vi "Generation Message Loop.vi"(8 "error in (no error)":errorcluster, 10 "Data Notifier":refnum<notifier>, 11 "Message Queues":T1) -> (0 "error out":errorcluster)   [LabVIEW 2014, in "PLS Generation.lvlib"]
doc: "Message loop for handling messages pertaining to the acquisition of data from the hardware."
uses:
  PLS Generation.lvlib
  support/Message Queue/All Message Queues.ctl
  support/Message Queue/Message Cluster.ctl
  Hardware Configuration.ctl
  Settings/conversion.ctl
  Generation State.ctl
  support/Message Queue/Enqueue Message (Single).vi
  <vilib>/Utility/error.llb/Error Cluster From Error Code.vi
  <vilib>/ErrorRing/Error Ring.xnode
  support/Message Queue/PLS Message Queue.lvlib
  Settings/PLS Settings.lvlib
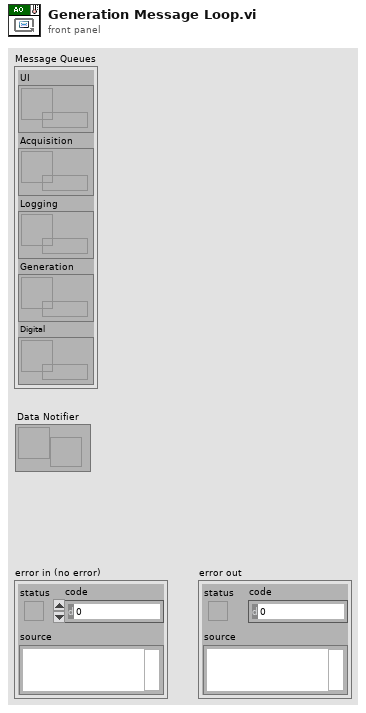
[diagram p1: front panel]
types:
  T1 = typedef "PLS Message Queue.lvlib/All Message Queues.ctl" = cluster{"UI":refnum<queue>, "Acquisition":refnum<queue>, "Logging":refnum<queue>, "Generation":refnum<queue>, "Digital":refnum<queue>}
  T2 = typedef "PLS Generation.lvlib/Hardware Configuration.ctl" = cluster{"AO":cluster{"task name":string, "task_ref":refnum<k21>, "physical channels":tag}, "PID":cluster{"P":dbl, "I":dbl, "D":dbl}, "conversions":cluster{"ao0":T3}, "setpoint":dbl}
  T3 = typedef "PLS Settings.lvlib/conversion.ctl" = cluster{"a":dbl, "b":dbl}
  T4 = typedef "PLS Generation.lvlib/Generation State.ctl" = enum16{"Idle", "Generate"}
  T5 = cluster{"task name":string, "task_ref":refnum<k21>, "physical channels":tag}
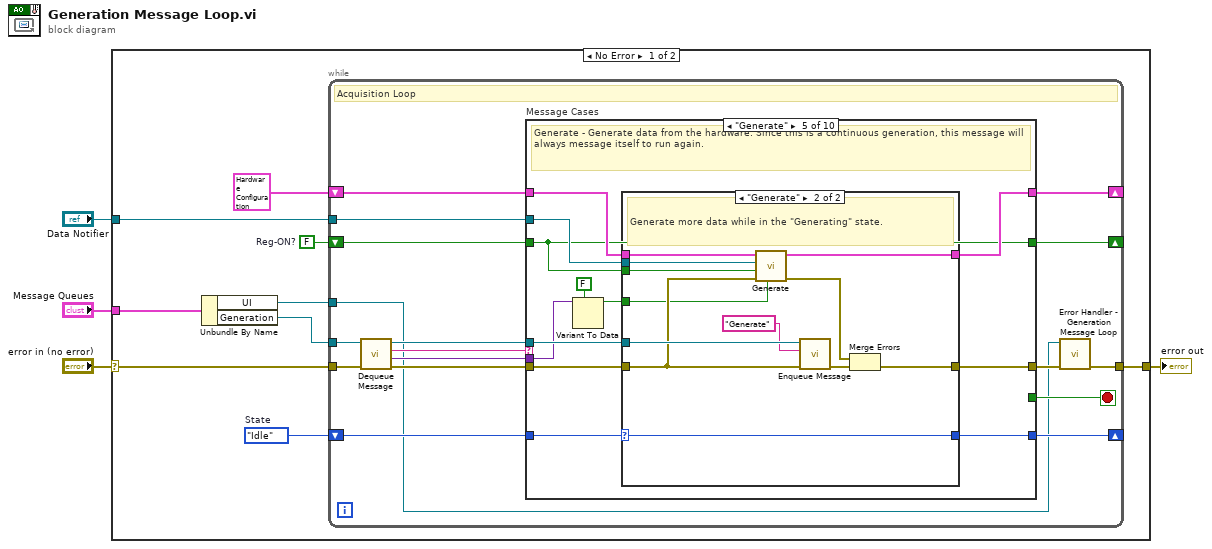
[diagram p0: block diagram]
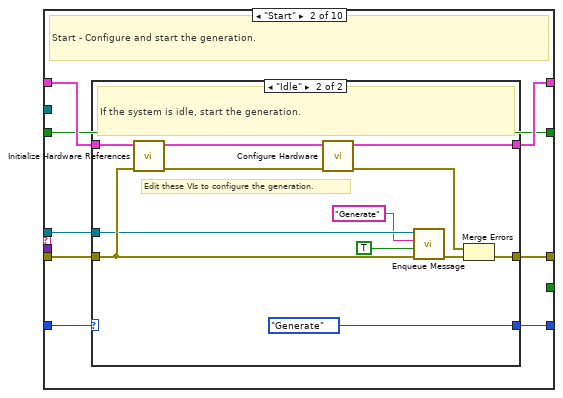
[diagram p3: hidden frame]
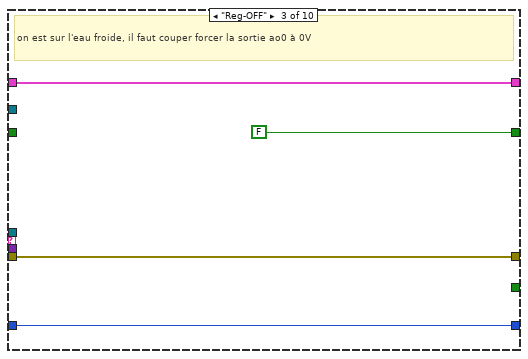
[diagram p5: hidden frame]
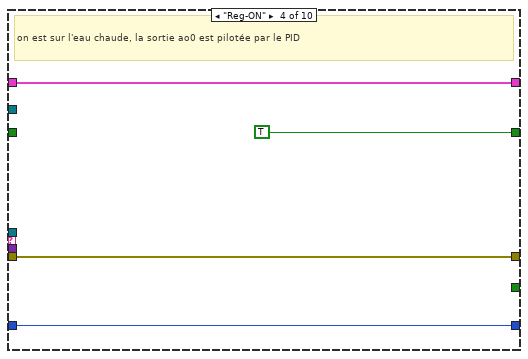
[diagram p6: hidden frame]
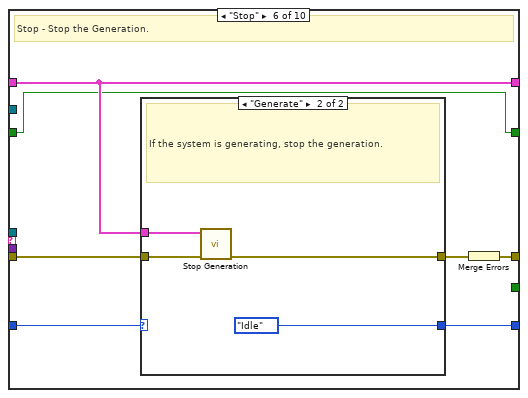
[diagram p8: hidden frame]
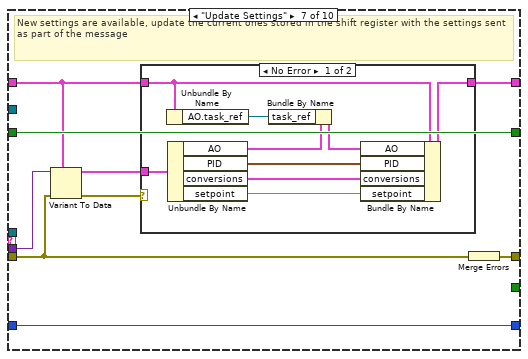
[diagram p10: hidden frame]
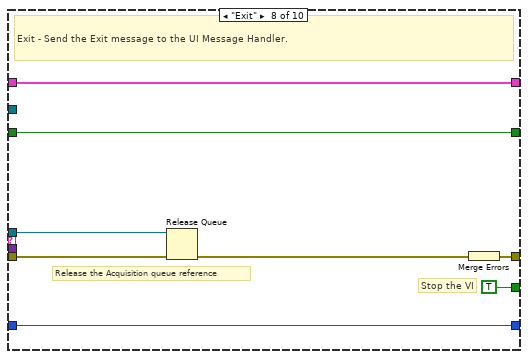
[diagram p12: hidden frame]
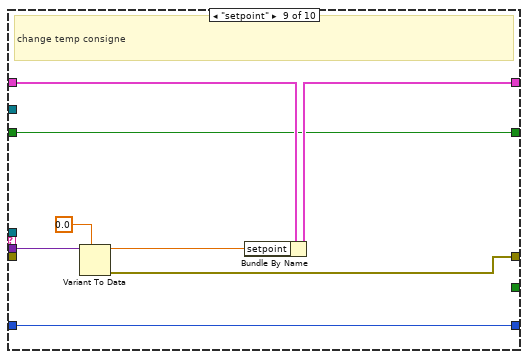
[diagram p13: hidden frame]
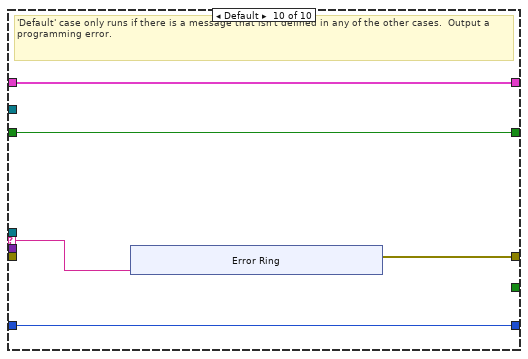
[diagram p14: hidden frame]
diagram:
  n1 = case shown="No Error" "error in (no error)" {
    selector: "error in (no error)" -> [w9 w153]
    tunnel: "Message Queues" -> [w13 _]
    tunnel: [w11 w153] -> w3
    tunnel: "Data Notifier" -> [w7 _]
    frame No Error {
      w5 = FALSE  # Reg-ON?
      w6 = Generation_State."Idle"  # State
      n2 = Unbundle By Name(w13) -> ("UI"=w8:refnum<queue>, "Generation"=w12:refnum<queue>)
      n3 = while {
        tunnel: w12 -> [w23]
        shift-right: [w29] -> _
        shift-left: T2 {"AO"={"task name"="AOO", "task_ref"="", "physical channels"="Dev1/ao0"}, "PID"={"P"=0.0, "I"=0.0, "D"=0.0}, "conversions"={"ao0"={"a"=1.0, "b"=0.0}}, "setpoint"=0.0} ("Data Cluster") -> [w30]
        tunnel: w8 -> [w16]
        tunnel: w7 -> [w22]
        shift-right: [w20] -> _
        shift-left: w6 -> [w21]
        tunnel: w9 -> [w27]
        tunnel: [w19] -> w11
        shift-right: [w15] -> _
        shift-left: w5 -> [w14]
        stop <- w28 stop-if-true
        # "Acquisition Loop"
        n4 = call "Dequeue Message.vi"("error in (no error)"=w27, "Message Queue"=w23) -> ("error out"=w26:errorcluster, "Message Data"=w24:variant, "Message"=w25:string, "dup Message Queue"=w17:refnum<queue>)  [unwired: 6 in]
        n5 = case "Message Cases" shown="\"Generate\"" w25 {
          selector: w25 -> [_ _ _ _ _ _ _ _ _ w142]
          tunnel: w17 -> [_ w39 _ _ w76 _ _ w127 _ _]
          tunnel: w26 -> [w34 w40 w59 w63 w75 w98 w111 w129 _ _]
          tunnel: [w34 w42 w59 w63 w77 w99 w114 w131 w134 w143] -> w18
          tunnel: w30 -> [w33 w41 w61 w65 w73 w96 w106 w130 w137 w145]
          tunnel: [w33 w38 w61 w65 w74 w96 w107 w130 w136 w145] -> w29
          tunnel: [_ _ _ _ _ _ _ TRUE _ _] -> w28
          tunnel: w24 -> [_ _ _ _ w68 _ w113 _ w139 _]
          tunnel: w22 -> [_ _ _ _ w72 _ _ _ _ _]
          tunnel: w21 -> [w32 w36 w60 w64 w70 w95 w110 w126 w140 w144]
          tunnel: [w32 w37 w60 w64 w71 w94 w110 w126 w140 w144] -> w20
          tunnel: [w31 w35 FALSE TRUE w69 w93 w109 w125 w133 w141] -> w15
          tunnel: w14 -> [w31 w35 _ _ w69 w93 w109 w125 w133 w141]
          frame "Initialize" {
            # "Initialize  - Initialize is currently a no-op.  The hardware initialization takes place in the 'Start' message."
          }
          frame "Start" {
            # "Start - Configure and start the generation."
            n6 = case shown="\"Idle\"" w36 {
              selector: w36 -> [w43 _]
              tunnel: [w44 w57] -> w42
              tunnel: w41 -> [w45 w56]
              tunnel: w40 -> [w44 w55]
              tunnel: w39 -> [_ w53]
              tunnel: [w45 w49] -> w38
              tunnel: [w43 Generation_State."Generate" ("Acquisition State")] -> w37
              frame "Generate" {
                # "The system is already generating. Ignore the \"Start\" message."
              }
              frame "Idle" {
                # "Edit these VIs to configure the generation."
                # "If the system is idle, start the generation."
                n7 = call "Initialize Hardware References.vi"("error in (no error)"=w55, "Hardware Resources in"=w56) -> ("error out"=w52:errorcluster, "Hardware Resources out"=w50:T2)  [unwired: 8 in]
                n8 = call "Configure Hardware.vi"("error in (no error)"=w52, "Hardware Resources in"=w50) -> ("error out"=w51:errorcluster, "Hardware Resources out"=w49:T2)  [unwired: 8 in]
                n9 = call-poly "Enqueue Message.vi"("error in (no error)"=w55, "Message Data"=TRUE, "Message"="Generate", "Message Queue"=w53) -> ("error out"=w54:errorcluster)  [unwired: 6 in, 1 out]
                n10 = Merge Errors(w51, w54) -> (w57:errorcluster)
              }
            }
          }
          frame "Reg-OFF" {
            # "on est sur l'eau froide, il faut couper forcer la sortie ao0 à 0V"
          }
          frame "Reg-ON" {
            # "on est sur l'eau chaude, la sortie ao0 est pilotée par le PID"
          }
          frame "Generate" {
            # "Generate - Generate data from the hardware. Since this is a continuous generation, this message will always message itself to run again."
            n11 = Variant To Data(type=FALSE ("reset"), Variant=w68) -> (data=w67:bool)  [unwired: 1 in, 1 out]
            n12 = case shown="\"Generate\"" w70 {
              selector: w70 -> [w78 w84]
              tunnel: [w79 w92] -> w77
              tunnel: w76 -> [_ w90]
              tunnel: w75 -> [w79 w83]
              tunnel: [w80 w88] -> w74
              tunnel: w73 -> [w80 w87]
              tunnel: w72 -> [_ w85]
              tunnel: [w78 w84] -> w71
              tunnel: w69 -> [_ w82]
              tunnel: w67 -> [_ w81]
              frame "Idle" {
                # "Ignore \"Generate\" messages when the generation is idle."
              }
              frame "Generate" {
                # "Generate more data while in the \"Generating\" state."
                n13 = call "Generate.vi"("reset"=w81, "error in (no error)"=w83, "Reg-ON?"=w82, "Data Notifier"=w85, "Hardware Resources in"=w87) -> ("error out"=w89:errorcluster, "Hardware Resources out"=w88:T2)  [unwired: 5 in]
                n14 = call-poly "Enqueue Message.vi"("error in (no error)"=w83, "Message"="Generate", "Message Queue"=w90) -> ("error out"=w91:errorcluster)  [unwired: 7 in, 1 out]
                n15 = Merge Errors(w89, w91) -> (w92:errorcluster)
              }
            }
          }
          frame "Stop" {
            # "Stop - Stop the Generation."
            n16 = case shown="\"Generate\"" w95 {
              selector: w95 -> [w100 _]
              tunnel: w98 -> [w101 w105]
              tunnel: [w101 w102] -> w97
              tunnel: w96 -> [_ w104]
              tunnel: [w100 Generation_State."Idle" ("State")] -> w94
              frame "Idle" {
                # "The system is already idle. Ignore the \"Stop\" message."
              }
              frame "Generate" {
                # "If the system is generating, stop the generation."
                n17 = call "Stop Generation.vi"("error in (no error)"=w105, "Hardware Resources in"=w104) -> ("error out"=w102:errorcluster)  [unwired: 9 in]
              }
            }
            n18 = Merge Errors(w97) -> (w99:errorcluster)
          }
          frame "Update Settings" {
            # "New settings are available, update the current ones stored in the shift register with the settings sent as part of the message"
            n19 = Variant To Data(error in=w111, type=w106, Variant=w113) -> (data=w112:T2, error out=w108:errorcluster)
            n20 = case shown="No Error" w108 {
              tunnel: w112 -> [w123 _]
              tunnel: w106 -> [w118 w124]
              tunnel: [w122 w124] -> w107
              frame No Error {
                n21 = Unbundle By Name(w118) -> ("AO.task_ref"=w117:refnum<k21>)
                n22 = Unbundle By Name(w123) -> ("AO"=w116:T5, "PID"=w121:cluster{"P":dbl, "I":dbl, "D":dbl}, "conversions"=w120:cluster{"ao0":T3}, "setpoint"=w119:dbl)
                n23 = Bundle By Name(cluster=w116, "task_ref"=w117) -> (w115:T5)
                n24 = Bundle By Name(cluster=w118, "AO"=w115, "PID"=w121, "conversions"=w120, "setpoint"=w119) -> (w122:T2)
              }
              frame Error {
              }
            }
            n25 = Merge Errors(w111) -> (w114:errorcluster)
          }
          frame "Exit" {
            # "Release the Acquisition queue reference"
            # "Stop the VI"
            # "Exit - Send the Exit message to the UI Message Handler."
            n26 = Release Queue(queue=w127, error in (no error)=w129) -> (error out=w128:errorcluster)  [unwired: 1 in, 2 out]
            n27 = Merge Errors(w128) -> (w131:errorcluster)
          }
          frame "setpoint" {
            # "change temp consigne"
            n28 = Variant To Data(type=0.0, Variant=w139) -> (data=w135:dbl, error out=w134:errorcluster)  [unwired: 1 in]
            n29 = Bundle By Name(cluster=w137, "setpoint"=w135) -> (w136:T2)
          }
          frame Default {
            # "'Default' case only runs if there is a message that isn't defined in any of the other cases.  Output a programming error."
            n30 = xnode "Error Ring"("parameter 0"=w142) -> ("error out"=w143:errorcluster)
          }
        }
        n31 = call "Error Handler - Generation Message Loop.vi"("error in (no error)"=w18, "Message Queue"=w16) -> ("dup error in"=w19:errorcluster)  [unwired: 8 in, 1 out]
      }
    }
    frame Error {
    }
  }
  "error out" <- w3
